vi "GetAvailableDeviceList.vi"(11 "Supported Devices":u32[](array[numeric])) -> (3 "Available Device List":u32[](array[numeric]))   [LabVIEW 2021, in "myRIOMetaDataObj.lvclass"]
uses:
  myRIOMetaDataObj.lvclass
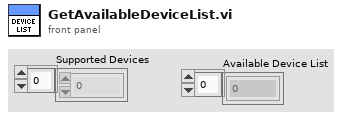
[diagram p1: front panel]
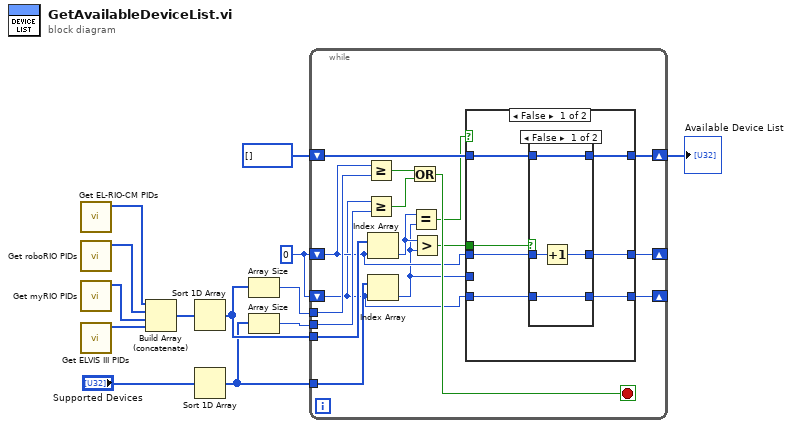
[diagram p0: block diagram]
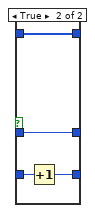
[diagram p2: hidden frame]
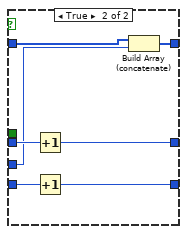
[diagram p3: hidden frame]
diagram:
  w8 = u32 0
  n1 = call <vilib>:"Get EL-RIO-CM PIDs.vi"() -> ("EL-RIO-CM PIDs"=w3:u32[])  [unwired: 11 in]
  n2 = call <vilib>:"Get roboRIO PIDs.vi"() -> ("roboRIO PIDs"=w2:u32[])  [unwired: 11 in]
  n3 = call <vilib>:"Get myRIO PIDs.vi"() -> ("myRIO PIDs"=w5:u32[])  [unwired: 11 in]
  n4 = call <vilib>:"Get ELVIS III PIDs.vi"() -> ("ELVIS III PIDs"=w1:u32[])  [unwired: 11 in]
  n5 = Build Array (concatenate)(w3, w2, w5, w1) -> (w4:u32[])
  n6 = Sort 1D Array(array=w4) -> (sorted array=w12:u32[])
  n7 = Sort 1D Array(array="Supported Devices") -> (sorted array=w10:u32[])
  n8 = Array Size(array=w12) -> (size(s)=w11:i32)
  n9 = Array Size(array=w10) -> (size(s)=w9:i32)
  n10 = while {
    tunnel: w10 -> [w24]
    tunnel: w12 -> [w25]
    tunnel: w11 -> [w30]
    tunnel: w9 -> [w29]
    shift-right: [w20] -> _
    shift-left: w8 -> [w19]
    shift-right: [w21] -> _
    shift-left: w8 -> [w18]
    shift-right: [w22] -> w7
    shift-left: u32[] [] -> [w23]
    stop <- w26 stop-if-true
    n11 = Greater Or Equal?(x=w19, y=w30) -> (x >= y?=w28:bool)
    n12 = Greater Or Equal?(x=w18, y=w29) -> (x >= y?=w27:bool)
    n13 = Index Array(array=w25, index=w19) -> (element=w16:u32)
    n14 = Index Array(array=w24, index=w18) -> (element=w15:u32)
    n15 = Or(x=w28, y=w27) -> (x .or. y?=w26:bool)
    n16 = Equal?(x=w16, y=w15) -> (x = y?=w17:bool)
    n17 = Greater?(x=w16, y=w15) -> (0:w14:bool)
    n18 = case shown="False" w17 {
      tunnel: w23 -> [w33 w52]
      tunnel: [w32 w51] -> w22
      tunnel: w19 -> [w37 w50]
      tunnel: w18 -> [w36 w48]
      tunnel: [w35 w47] -> w21
      tunnel: [w34 w49] -> w20
      tunnel: w15 -> [_ w46]
      tunnel: w14 -> [w31 _]
      frame False {
        n19 = case shown="False" w31 {
          tunnel: w37 -> [w40 w43]
          tunnel: w36 -> [w38 w45]
          tunnel: [w38 w44] -> w35
          tunnel: [w39 w43] -> w34
          tunnel: w33 -> [w41 w42]
          tunnel: [w41 w42] -> w32
          frame False {
            n20 = Increment(x=w40) -> (x+1=w39:u32)
          }
          frame True {
            n21 = Increment(x=w45) -> (x+1=w44:u32)
          }
        }
      }
      frame True {
        n22 = Increment(x=w50) -> (x+1=w49:u32)
        n23 = Increment(x=w48) -> (x+1=w47:u32)
        n24 = Build Array (concatenate)(w52, w46) -> (w51:u32[])
      }
    }
  }
  "Available Device List" <- w7
